vi "Control_Save_or_Load.vi"() -> ()   [LabVIEW 2023]
uses:
  <vilib>/Utility/sysdir.llb/System Directory Type.ctl
panel:
  out "File Path":path
  in  "Exit":bool
  in  "Load":bool
  in  "Save":bool
  in  "String":string
  out "Boolean":bool
  in  "Numeric":dbl
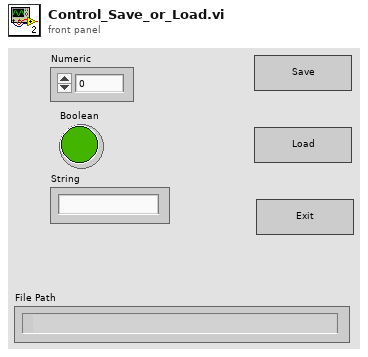
[diagram p1: front panel]
types:
  T1 = typedef "System Directory Type.ctl" = i32
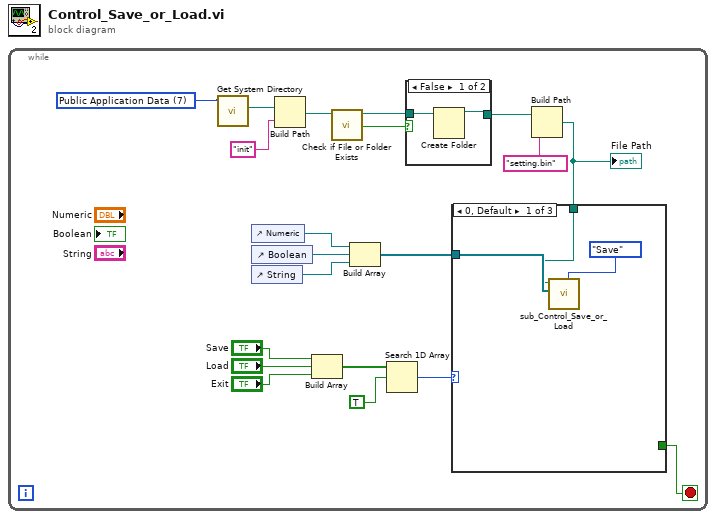
[diagram p0: block diagram]
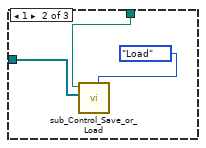
[diagram p3: hidden frame]
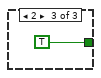
[diagram p4: hidden frame]
diagram:
  n1 = while {
    stop <- w2 stop-if-true
    w14 = T1 7 items=["User Home"=0, "User Desktop"=1, "User Documents"=2, "User Application Data"=3, "User Preferences"=4, "User Temporary"=5, "Public Documents"=6, "Public Application Data"=7, "Public Preferences"=8, "Public Cache"=13, "System Core Libraries"=9, "System Installed Libraries"=10, "Application Files"=11, "Boot Volume Root"=12] ("system directory type")
    n2 = call <vilib>:"Get System Directory.vi"("system directory type"=w14) -> ("system directory"=w13:path)  [unwired: 10 in]
    n3 = control-ref of="Numeric"() -> (w5:refnum<vi>)
    n4 = control-ref of="Boolean"() -> (w6:refnum<vi>)
    n5 = control-ref of="String"() -> (w4:refnum<vi>)
    n6 = Build Path(base path=w13, name or relative path="init") -> (appended path=w11:path)
    n7 = Build Array("Save", "Load", "Exit") -> (w17:bool[])
    n8 = call <vilib>:"Check if File or Folder Exists.vi"("path"=w11) -> ("file or folder exists?"=w10:bool, "dup path"=w9:path)  [unwired: 8 in, 1 out]
    n9 = Build Array(w5, w6, w4) -> (w3:refnum<vi>[])
    n10 = Search 1D Array(1D array=w17, element=TRUE) -> (index of element=w15:i32)  [unwired: 1 in]
    n11 = case shown="False" w10 {
      tunnel: w9 -> [w22 w23]
      tunnel: [w21 w23] -> w8
      frame False {
        n12 = Create Folder(path (use dialog)=w22) -> (created path=w21:path)  [unwired: 2 in, 2 out]
      }
      frame True {
      }
    }
    n13 = Build Path(base path=w8, name or relative path="setting.bin") -> (appended path=w1:path)
    "File Path" <- w1
    n14 = case shown="0, Default" w15 {
      tunnel: w3 -> [w26 w28 _]
      tunnel: w1 -> [w25 w27 _]
      tunnel: [_ _ TRUE] -> w2
      frame 0, Default {
        n15 = call "sub_Control_Save_or_Load.vi"("Enum"=enum16{"Save", "Load"}."Save", "Array"=w26, "File Path"=w25) -> ()  [unwired: 8 in, 1 out]
      }
      frame 1 {
        n16 = call "sub_Control_Save_or_Load.vi"("Enum"=enum16{"Save", "Load"}."Load", "Array"=w28, "File Path"=w27) -> ()  [unwired: 8 in, 1 out]
      }
      frame 2 {
      }
    }
  }
